vi "Plotting Main.vi"() -> ()   [LabVIEW 2016]
uses:
  Refrigeration/RTS/Type Definitions/RTS TDMS Filename Locations.ctl
panel:
  in  "TDMS Data Save":T1
  in  "Debug?":bool
  out "Debug array":string[](array[string])
  in  "Update Plot":bool
  out "Button":u16
  in  "OK":bool
  in  "Multicolumn Listbox":i32[](listbox)
  out "Mixed Signal Graph":T2(graph)
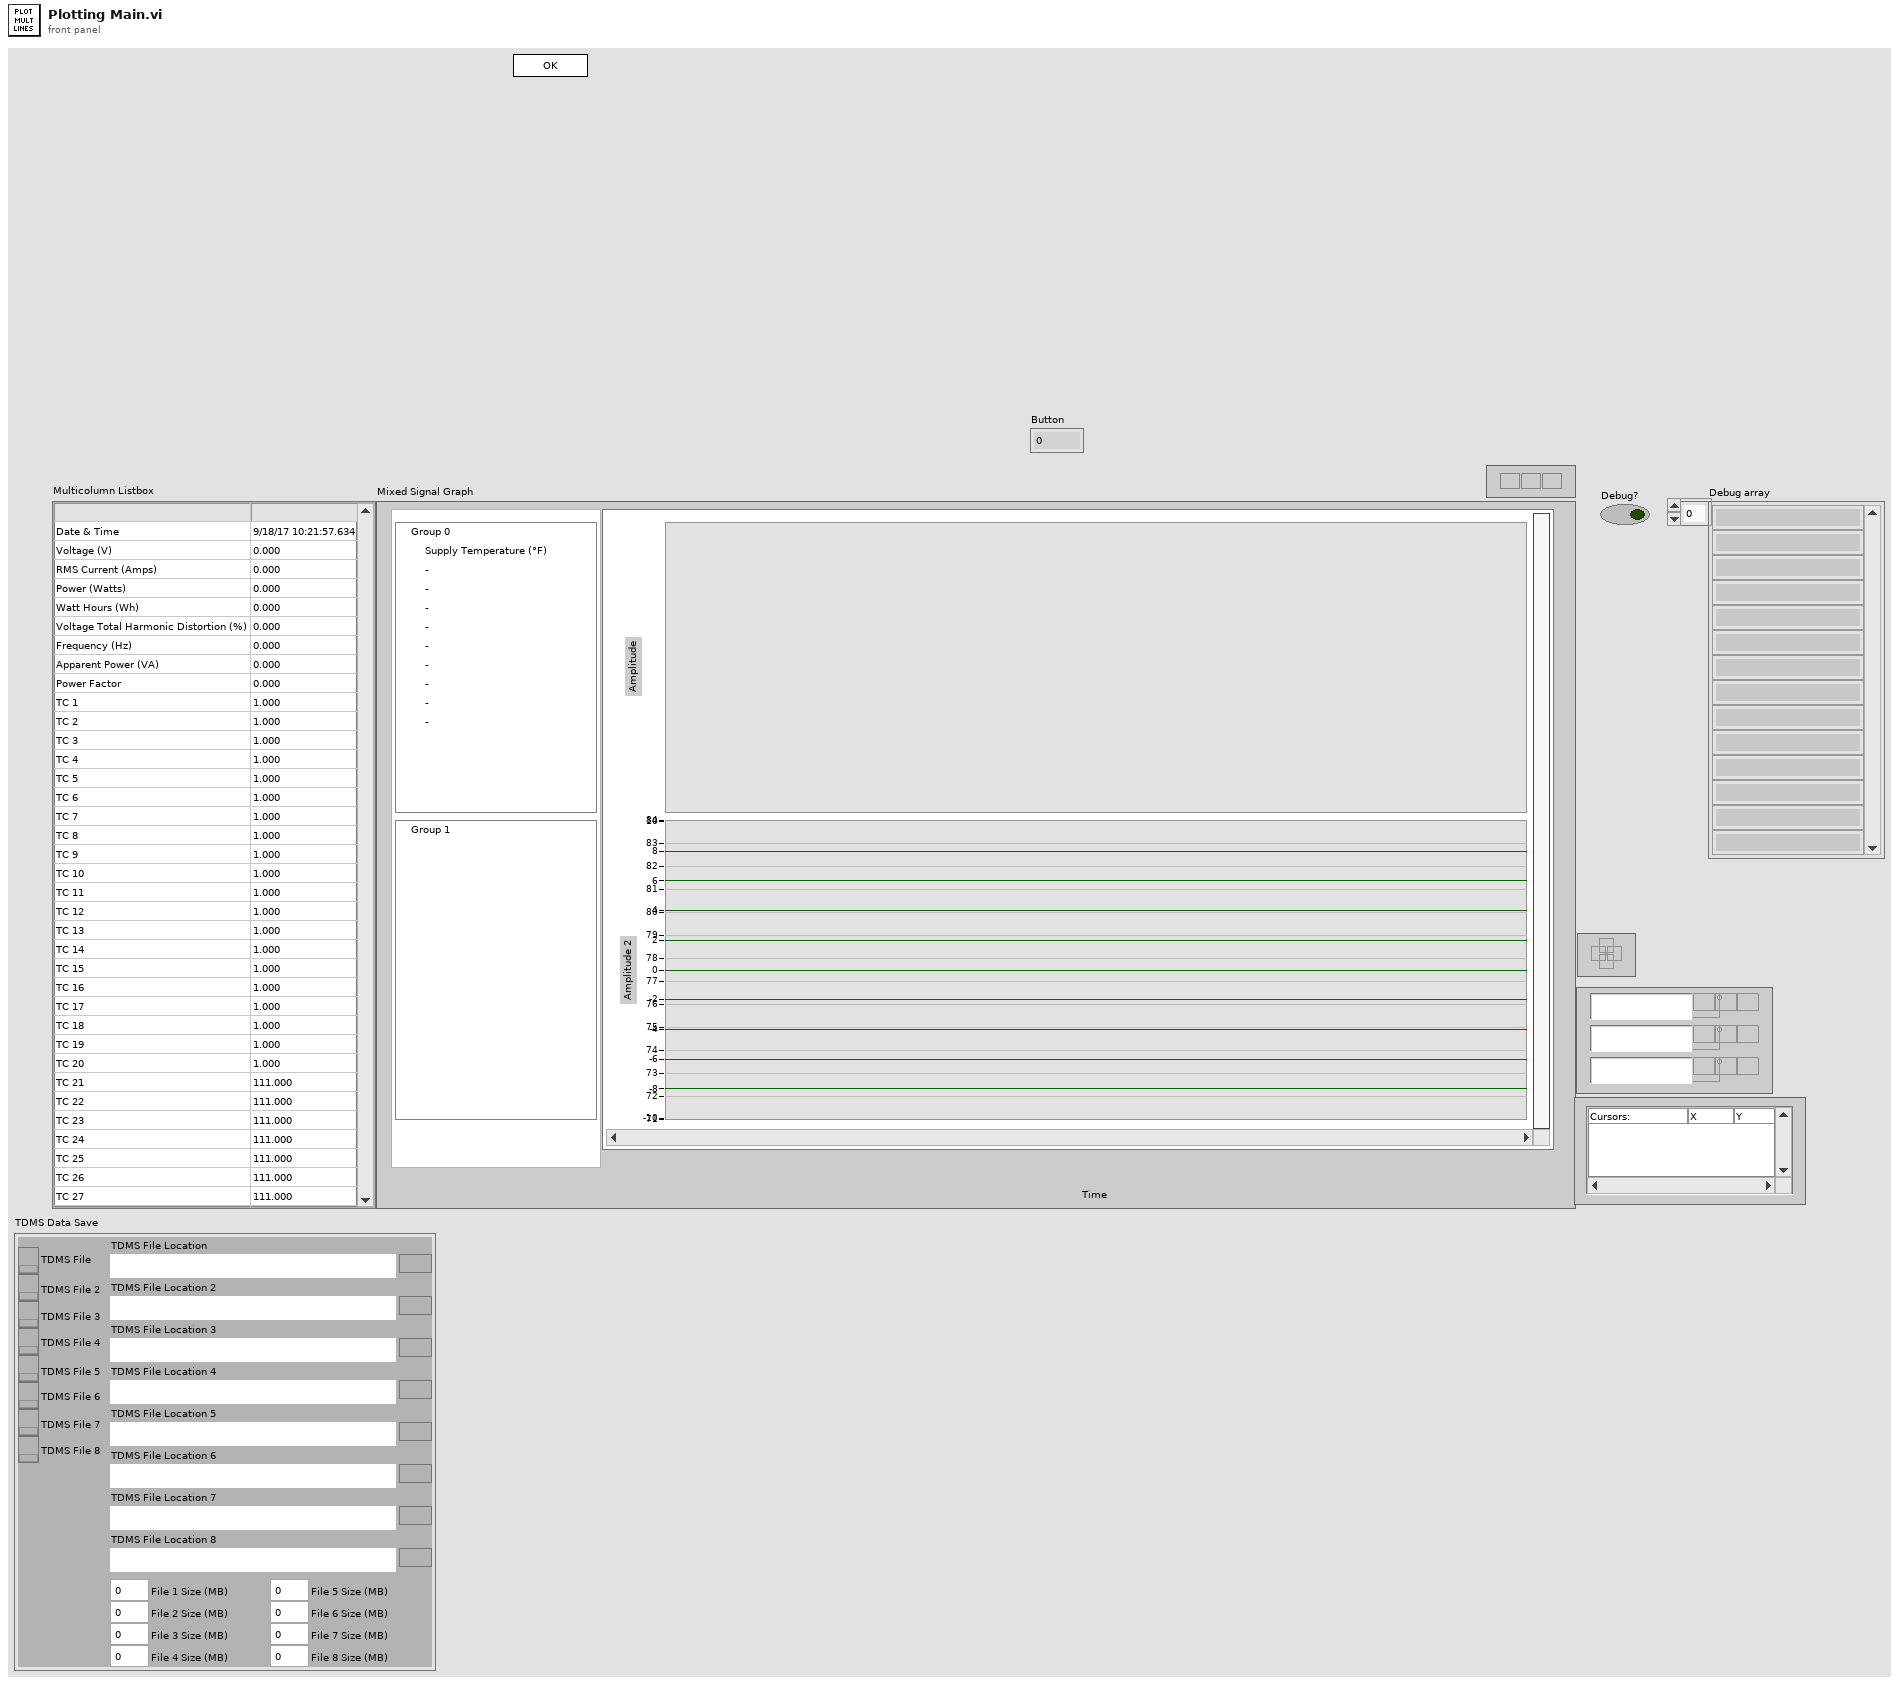
[diagram p1: front panel]
types:
  T1 = typedef "RTS TDMS Filename Locations.ctl" = cluster{"TDMS File":refnum<k34>, "TDMS File Location":path, "TDMS File Location 2":path, "TDMS File Location 3":path, "TDMS File Location 4":path, "TDMS File Location 5":path, "TDMS File Location 6":path, "TDMS File Location 7":path, "TDMS File Location 8":path, "TDMS File 2":refnum<k34>, "TDMS File 3":refnum<k34>, "TDMS File 4":refnum<k34>, "TDMS File 5":refnum<k34>, "TDMS File 6":refnum<k34>, "TDMS File 7":refnum<k34>, "TDMS File 8":refnum<k34>, "File 1 Size (MB)":dbl, "File 2 Size (MB)":dbl, "File 3 Size (MB)":dbl, "File 4 Size (MB)":dbl, "File 5 Size (MB)":dbl, "File 6 Size (MB)":dbl, "File 7 Size (MB)":dbl, "File 8 Size (MB)":dbl}
  T2 = cluster{"Waveform Graph":waveform(dbl), "Waveform Graph":waveform(dbl), "Waveform Graph":waveform(dbl), "Waveform Graph":waveform(dbl), "Waveform Graph":waveform(dbl), "Waveform Graph":waveform(dbl), "Waveform Graph":waveform(dbl), "Waveform Graph":waveform(dbl), "Waveform Graph":waveform(dbl), "Waveform Graph":waveform(dbl)}
  T3 = enum32{"invalid app kind", "Development System", "Run Time System", "Student Edition", "Embedded LabVIEW", "Evaluation", "Custom"}
  T4 = enum32{"Invalid", "Standard", "Closed", "Hidden", "Minimized", "Maximized"}
  T5 = cluster{"Core":cluster{"Current VI Reference":refnum<vi>, "Close Panel on Exit?":bool}, "ListBox Selection":i32[], "All Data":dbl[][], "Item Names":string[], "TDMS Data Save":T1}
  T6 = cluster{"Current VI Reference":refnum<vi>, "Close Panel on Exit?":bool}
  T7 = typedef "RTS TDMS Data.ctl" = cluster{"Station 1":dbl[][], "Station 2":dbl[][], "Station 3":dbl[][], "Station 4":dbl[][], "Station 5":dbl[][], "Station 6":dbl[][], "Station 7":dbl[][], "Station 8":dbl[][]}
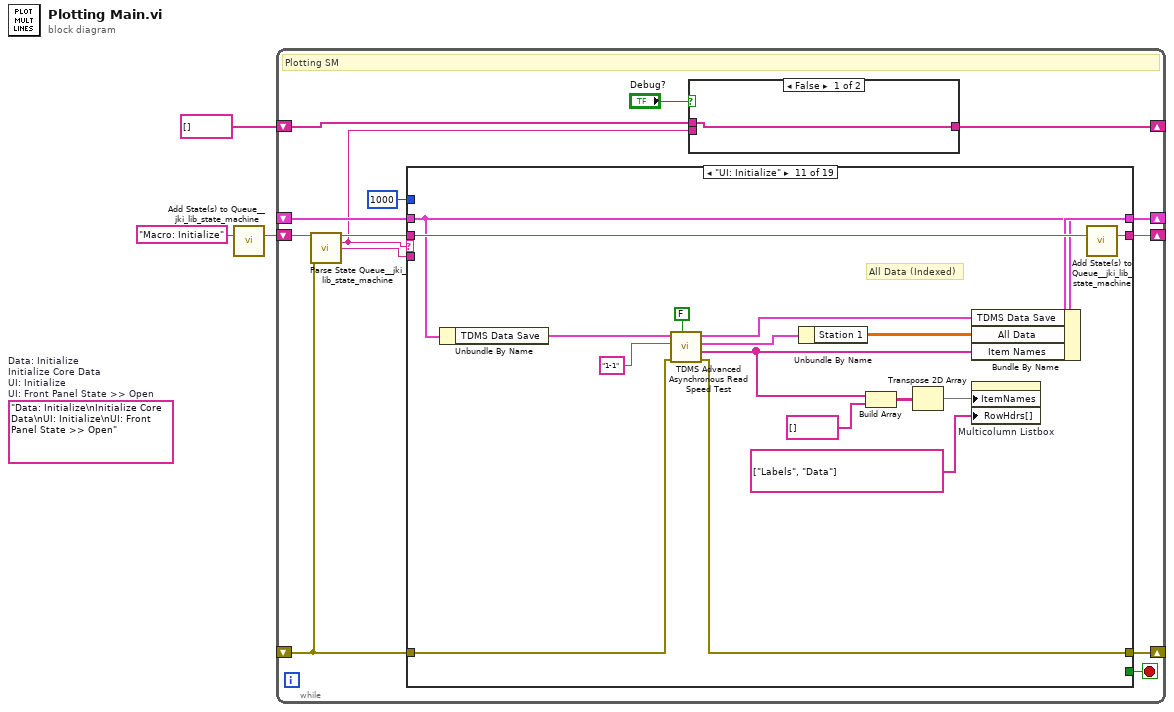
[diagram p0: block diagram]
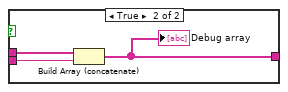
[diagram p2: hidden frame]
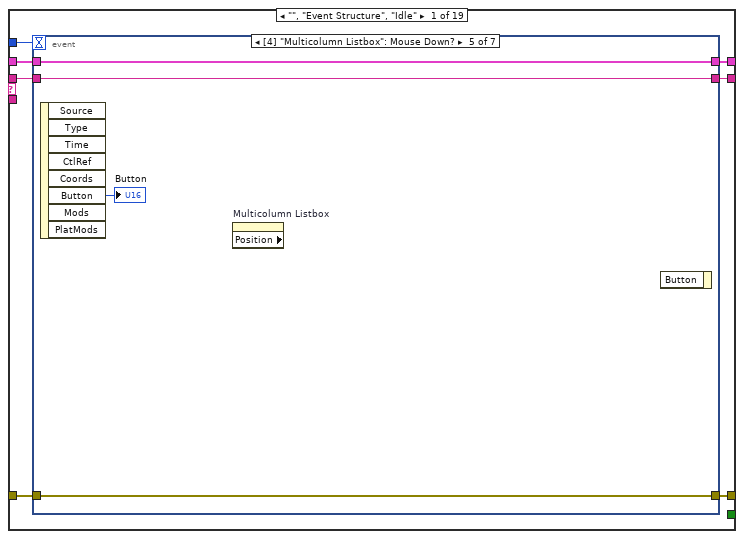
[diagram p3: hidden frame]
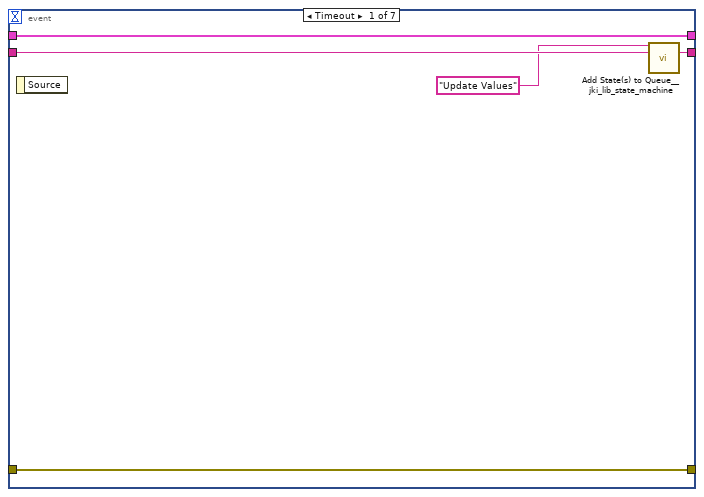
[diagram p4: hidden frame]
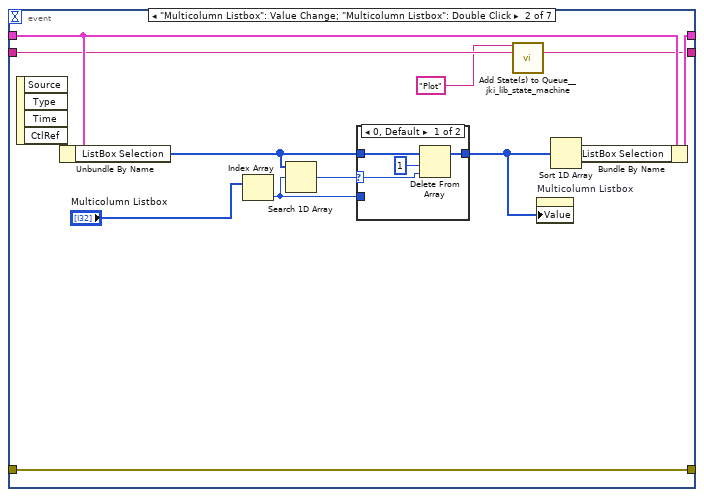
[diagram p5: hidden frame]
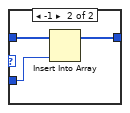
[diagram p6: hidden frame]
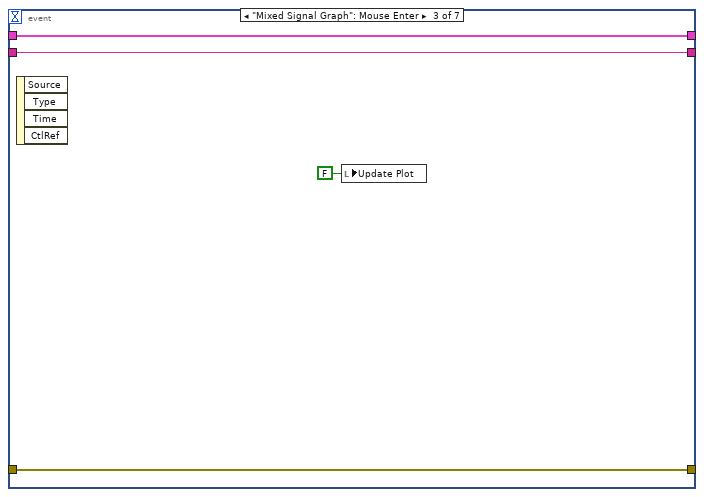
[diagram p7: hidden frame]
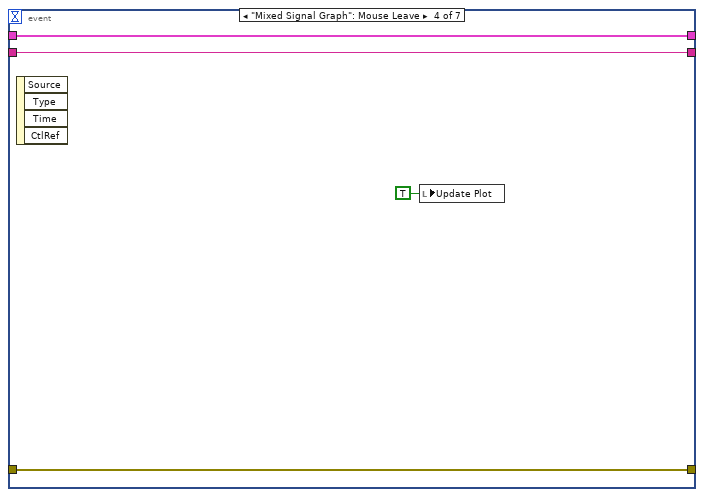
[diagram p8: hidden frame]
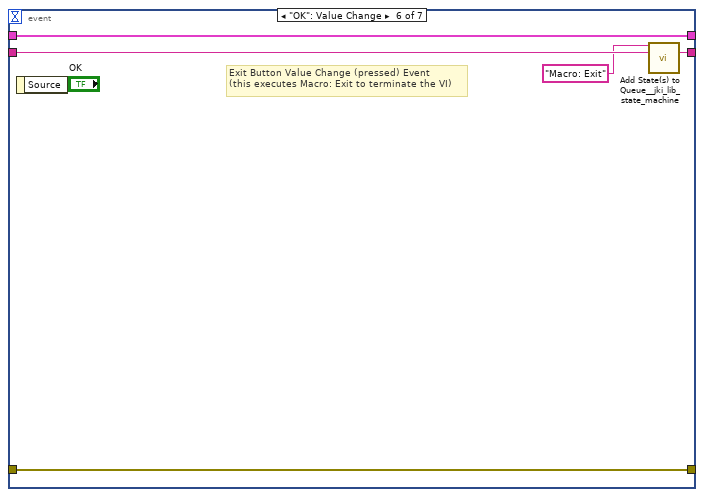
[diagram p9: hidden frame]
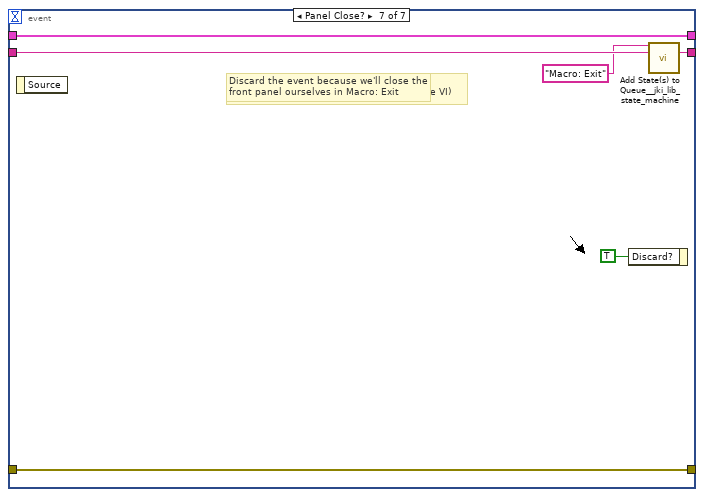
[diagram p10: hidden frame]
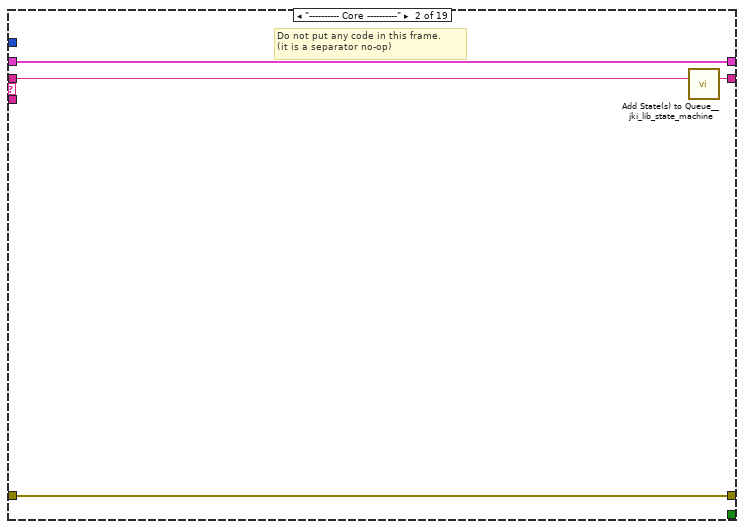
[diagram p11: hidden frame]
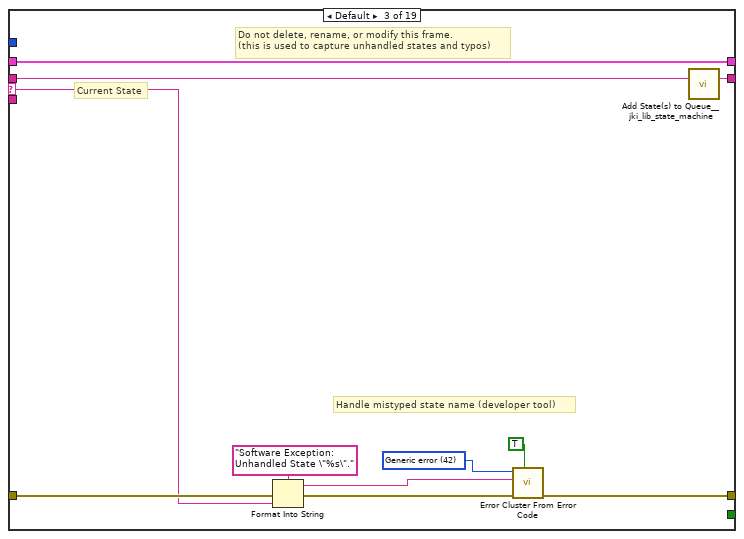
[diagram p12: hidden frame]
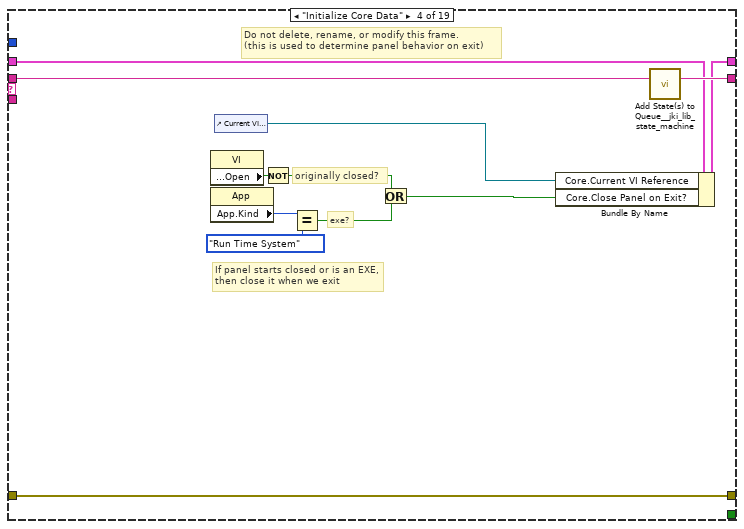
[diagram p13: hidden frame]
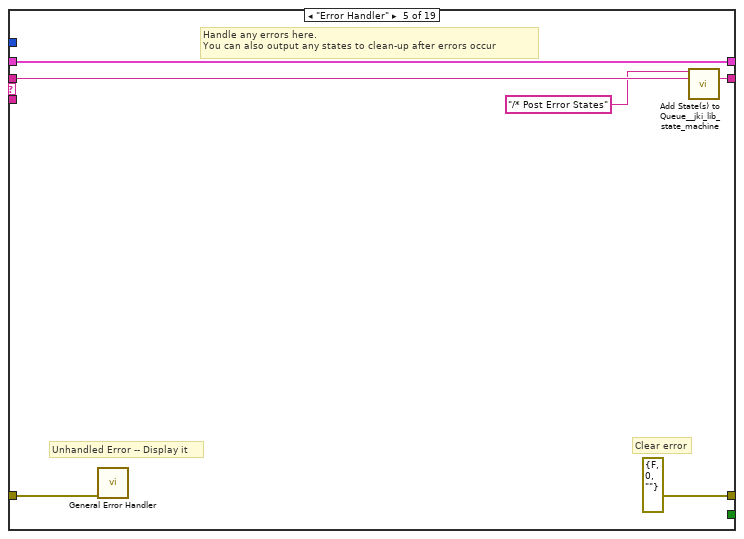
[diagram p14: hidden frame]
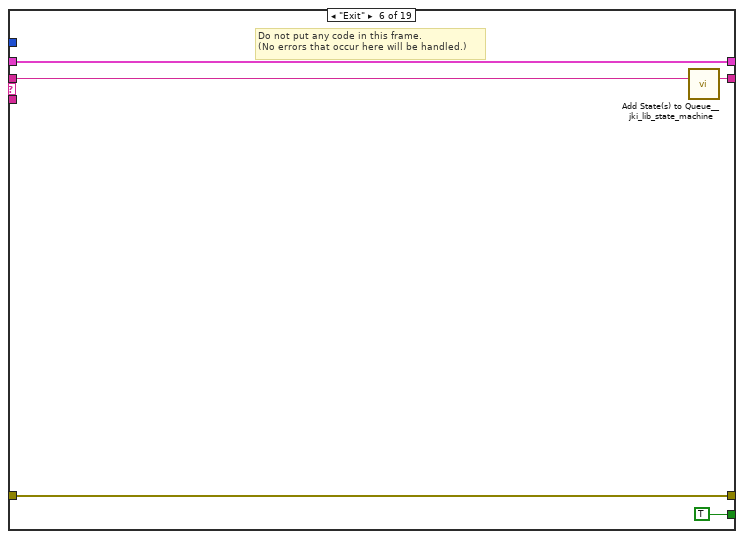
[diagram p15: hidden frame]
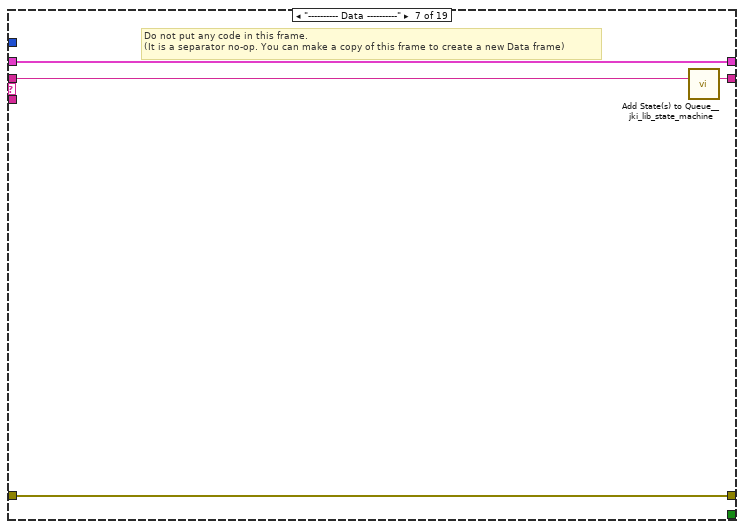
[diagram p16: hidden frame]
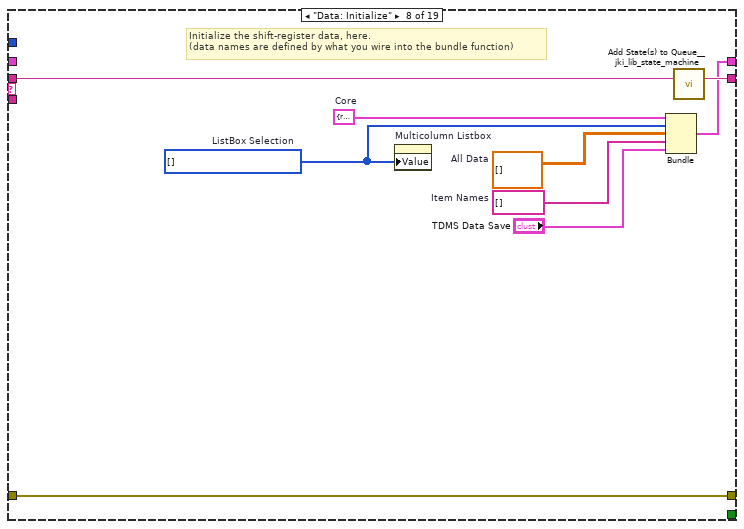
[diagram p17: hidden frame]
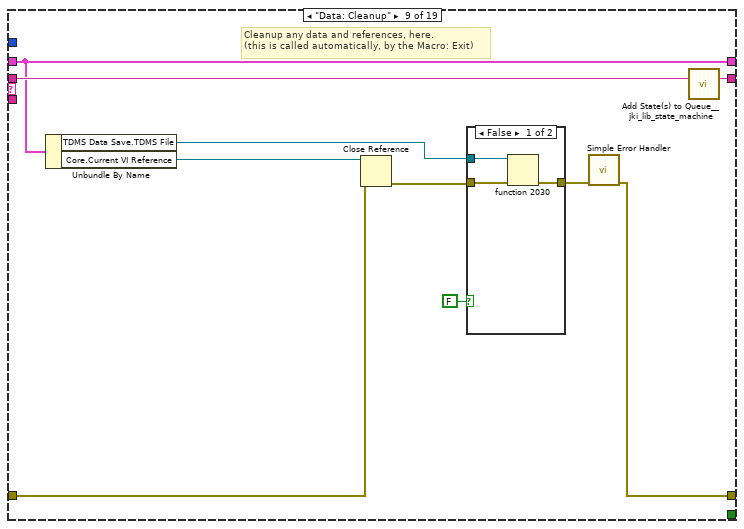
[diagram p18: hidden frame]
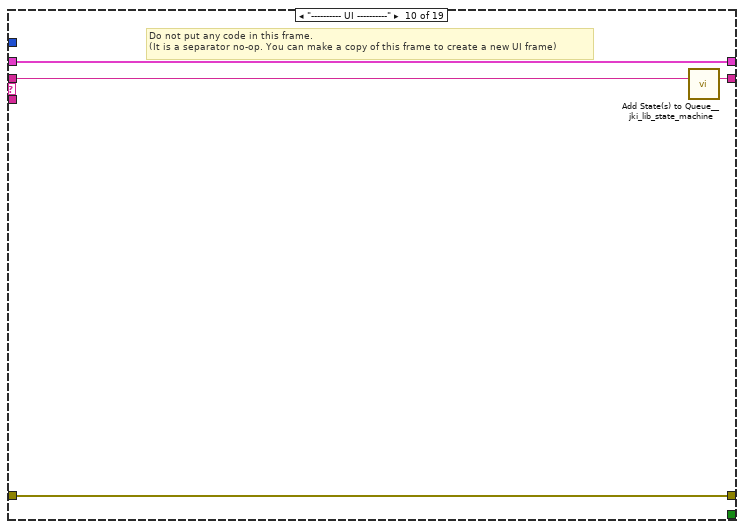
[diagram p20: hidden frame]
diagram:
  (unwired) "Data: Initialize\nInitialize Core Data\nUI: Initialize\nUI: Front Panel State >> Open"  # Data: Initialize Initialize Core Data UI: Initialize UI: Front Panel State >> Open
  n1 = call <vilib>:"Add State(s) to Queue__jki_lib_state_machine.vi"("State(s) in (\"\")"="Macro: Initialize") -> ("States Out"=w3:string)  [unwired: 14 in]
  n2 = while "Plotting SM" {
    shift-right: [w11] -> _
    shift-left: _ -> [w10]
    shift-right: [w14] -> _
    shift-left: _ -> [w8]
    shift-right: [w13] -> _
    shift-left: w3 -> [w15]
    shift-right: [w5] -> _
    shift-left: string[] [] -> [w7]
    stop <- w12 stop-if-true
    # "Plotting SM"
    n3 = call <vilib>:"Parse State Queue__jki_lib_state_machine.vi"("State Queue"=w15, "Error In (no error)"=w8) -> ("Remaining States"=w17:string, "Current State"=w6:string, "Arguments"=w16:string)  [unwired: 11 in]
    n4 = case shown="\"UI: Initialize\"" w6 {
      selector: w6 -> [_ _ w80 _ _ _ _ _ _ _ _ _ _ _ _ _ _ _ _]
      tunnel: w17 -> [w28 w79 w84 w102 w108 w113 w117 w126 w136 w144 w161 w167 w178 w204 w209 w219 w223 w231 w253]
      tunnel: w16 -> [_ _ _ _ _ _ _ _ _ _ _ w162 w172 _ _ _ _ _ _]
      tunnel: w10 -> [w26 w76 w82 w93 w105 w111 w114 _ w132 w141 w153 w165 w174 w201 w206 w216 w220 w228 w236]
      tunnel: [w25 w77 w86 w99 errorcluster {"status"=FALSE, "code"=0, "source"=""} ("error out") w110 w115 w123 w129 w142 w145 w163 w175 w202 w207 w217 w221 w229 w237] -> w14
      tunnel: w8 -> [w24 w77 w85 w99 w104 w110 w115 w123 w133 w142 w146 w164 w176 w202 w207 w217 w221 w229 w247]
      tunnel: [w27 w78 w83 w101 w107 w112 w116 w125 w135 w143 w160 w166 w177 w203 w208 w218 w222 w230 w252] -> w13
      tunnel: [_ _ _ _ _ TRUE _ _ _ _ _ _ _ _ _ _ _ _ _] -> w12
      tunnel: [w23 w76 w82 w100 w105 w111 w114 w124 w132 w141 w159 w165 w174 w201 w206 w216 w220 w228 w250] -> w11
      tunnel: 1000 ("Timeout") -> [w22 _ _ _ _ _ _ _ _ _ _ _ _ _ _ _ _ _ _]
      frame "", "Event Structure", "Idle" {
        n5 = event shown="[4] \"Multicolumn Listbox\": Mouse Down?" {
          selector: _ -> [_ _ _ _ _ _ _]
          dyn-events: _ -> [_ _ _ _ _ _ _]
          timeout: w22 -> [_ _ _ _ _ _ _]
          tunnel: w28 -> [w33 w38 w55 w59 w62 w69 w75]
          tunnel: [w32 w37 w55 w59 w62 w68 w74] -> w27
          tunnel: w26 -> [w30 w44 w56 w58 w63 w66 w72]
          tunnel: [w31 w45 w54 w60 w64 w67 w73] -> w25
          tunnel: w24 -> [w31 w45 w54 w60 w64 w67 w73]
          tunnel: [w30 w43 w56 w58 w63 w66 w72] -> w23
          event Timeout {
            n6 = event-data() -> ()  [unwired: 1 in, 1 out]
            n7 = call <vilib>:"Add State(s) to Queue__jki_lib_state_machine.vi"("State(s) in Front (\"\")"="Update Values" ("State(s) in Front (\"\")"), "State(s) in (\"\")"=w33) -> ("States Out"=w32:string)  [unwired: 13 in]
          }
          event "Multicolumn Listbox": Value Change; "Multicolumn Listbox": Double Click {
            n8 = event-data() -> ()  [unwired: 1 in, 4 out]
            n9 = Unbundle By Name(w44) -> ("ListBox Selection"=w39:i32[])
            n10 = Index Array(array="Multicolumn Listbox") -> (element=w41:i32)  [unwired: 1 in]
            n11 = Search 1D Array(1D array=w39, element=w41) -> (index of element=w40:i32)  [unwired: 1 in]
            n12 = case shown="0, Default" w40 {
              selector: w40 -> [w46 _]
              tunnel: w41 -> [_ w52]
              tunnel: w39 -> [w49 w51]
              tunnel: [w48 w50] -> w35
              frame 0, Default {
                n13 = Delete From Array(array=w49, length=1, index=w46) -> (array with subset deleted=w48:i32[])  [unwired: 1 out]
              }
              frame -1 {
                n14 = Insert Into Array(array=w51, new element=w52) -> (w50:i32[])  [unwired: 1 in]
              }
            }
            n15 = call <vilib>:"Add State(s) to Queue__jki_lib_state_machine.vi"("State(s) in Front (\"\")"="Plot" ("State(s) in Front (\"\")"), "State(s) in (\"\")"=w38) -> ("States Out"=w37:string)  [unwired: 13 in]
            n16 = property on="Multicolumn Listbox" class="MCListbox (strict)"("Value"=w35) -> ()  [unwired: 2 in, 2 out]
            n17 = Sort 1D Array(array=w35) -> (sorted array=w34:i32[])
            n18 = Bundle By Name(cluster=w44, "ListBox Selection"=w34) -> (w43:T5)
          }
          event "Mixed Signal Graph": Mouse Enter {
            n19 = event-data() -> ()  [unwired: 1 in, 4 out]
            n20 = local write "Update Plot"(FALSE ("Update Plot")) -> ()
          }
          event "Mixed Signal Graph": Mouse Leave {
            n21 = event-data() -> ()  [unwired: 1 in, 4 out]
            n22 = local write "Update Plot"(TRUE ("Update Plot")) -> ()
          }
          event "Multicolumn Listbox": Mouse Down? {
            n23 = event-data() -> ("Button"=→"Button":u16)  [unwired: 1 in, 7 out]
            n24 = property on="Multicolumn Listbox" class="MCListbox (strict)" props=["Position"]() -> ()  [unwired: 2 in, 3 out]
            n25 = event-data() -> ()  [unwired: 2 in, 1 out]
          }
          event "OK": Value Change {
            # "Exit Button Value Change (pressed) Event\n(this executes Macro: Exit to terminate the VI)"
            n26 = event-data() -> ()  [unwired: 1 in, 1 out]
            n27 = call <vilib>:"Add State(s) to Queue__jki_lib_state_machine.vi"("State(s) in Front (\"\")"="Macro: Exit", "State(s) in (\"\")"=w69) -> ("States Out"=w68:string)  [unwired: 13 in]
          }
          event Panel Close? {
            # "Discard the event because we'll close the front panel ourselves in Macro: Exit"
            # "Close Panel button (pressed) Event\n(this executes Macro: Exit to terminate the VI)"
            n28 = event-data() -> ()  [unwired: 1 in, 1 out]
            n29 = event-data("Discard?"=TRUE) -> ()  [unwired: 1 in, 1 out]
            n30 = call <vilib>:"Add State(s) to Queue__jki_lib_state_machine.vi"("State(s) in Front (\"\")"="Macro: Exit", "State(s) in (\"\")"=w75) -> ("States Out"=w74:string)  [unwired: 13 in]
          }
        }
      }
      frame "---------- Core ----------" {
        # "Do not put any code in this frame.\n(it is a separator no-op)"
        n31 = call <vilib>:"Add State(s) to Queue__jki_lib_state_machine.vi"("State(s) in (\"\")"=w79) -> ("States Out"=w78:string)  [unwired: 14 in]
      }
      frame Default {
        w89 = 42 items=["No error", "Argument error", "Memory is full", "Out of zone", "End of file", "File already open", "Generic file I/O error", "File not found", "File permission error", "Disk is full", "Duplicate path", "Too many files open", "System feature not enabled", "Resource file not found", "Cannot add resource", "Resource not found", "Image not found", "Image memory error", "Pen does not exist", "Config type invalid", "Config token not found", "Config parse error", "Config memory error", "Bad external code format", "Bad external code offset", "External code not present", "Null window", "Destroy window error", "Null menu", "Print aborted", "Bad print record", "Print driver error", "Windows error during printing", "Memory error during printing", "Print dialog error", "Generic print error", "Invalid device refnum", "Device not found", "Device parameter error", "Device unit error", "Cannot open device", "Device call aborted", "Generic error", "Cancelled by user", "Object ID too low", "Object ID too high", "Object not in heap", "Unknown heap", "Unknown object (invalid DefProc)", "Unknown object (DefProc not in table)", "Message out of range", "Invalid (null) method", "Unknown message", "Manager call not supported", "Bad address", "Network operation in progress", "Network operation timed out", "Connection is busy", "Network attribute not supported", "Network error", "Address in use", "System out of memory", "Connection aborted", "Connection refused", "Not connected", "Already connected", "Connection closed", "Initialization error (interapplication manager)", "Bad occurrence", "Wait on unbound occurrence handler", "Occurrence queue overflow", "Datalog type conflict", "Unused", "Unrecognized type (interapplication manager)", "Memory corrupt", "Failed to make temporary DLL", "Old CIN version", "Drag socket not found", "Failed to load drop-object", "Failed to register OLE object", "Failed to release OLE object", "Format specifier type mismatch", "Unknown format specifier", "Too few format specifiers", "Too many format specifiers", "Scan failed", "Newer CIN version", "Error converting to variant", "Runtime menu error", "Password tampered", "Variant attribute not found", "Incompatible variant data type", "Event data is not available", "Event Store is not present", "Occurrence is not found", "Event Queue is not created", "Event info is not available", "Refnum passed is NULL", "Error retrieving Class GUID", "Error retrieving CoClass GUID", "Error retrieving TypeLib GUID.", "Bad built application magic bytes.", "Specific driver is different from the specific driver associated with the Logical Name.", "There is no session opened to the class driver.", "Max Error", "MAX - Error with config objects", "MAX - Error loading configuration", "MAX - Group not supported"]
        # "Current State"
        # "Do not delete, rename, or modify this frame.\n(this is used to capture unhandled states and typos)"
        # "Handle mistyped state name (developer tool)"
        n32 = Format Into String(format string="Software Exception: Unhandled State \"%s\"." ("message"), error in=w85, w80) -> (resulting string=w88:string, error out=w87:errorcluster)  [unwired: 1 in]
        n33 = call <vilib>:"Error Cluster From Error Code.vi"("show call chain? (False)"=TRUE, "error in (no error)"=w87, "error message (\"\")"=w88, "error code (0)"=w89) -> ("error out"=w86:errorcluster)  [unwired: 5 in]
        n34 = call <vilib>:"Add State(s) to Queue__jki_lib_state_machine.vi"("State(s) in (\"\")"=w84) -> ("States Out"=w83:string)  [unwired: 14 in]
      }
      frame "Initialize Core Data" {
        # "Do not delete, rename, or modify this frame.\n(this is used to determine panel behavior on exit)"
        # "originally closed?"
        # "exe?"
        # "If panel starts closed or is an EXE, then close it when we exit"
        n35 = property class="VI"() -> ("Front Panel.Open"=w98:bool)  [unwired: 2 in, 2 out]
        n36 = property class="App"() -> ("App.Kind"=w97:T3)  [unwired: 2 in, 2 out]
        n37 = control-ref of="Current VI Reference"() -> (w91:refnum<vi>)
        n38 = Not(x=w98) -> (.not. x?=w95:bool)
        n39 = Equal?(x=w97, y=T3."Run Time System" ("Application:Kind")) -> (x = y?=w94:bool)
        n40 = Or(x=w95, y=w94) -> (x .or. y?=w92:bool)
        n41 = Bundle By Name(cluster=w93, "Core.Current VI Reference"=w91, "Core.Close Panel on Exit?"=w92) -> (w100:T5)
        n42 = call <vilib>:"Add State(s) to Queue__jki_lib_state_machine.vi"("State(s) in (\"\")"=w102) -> ("States Out"=w101:string)  [unwired: 14 in]
      }
      frame "Error Handler" {
        # "Unhandled Error -- Display it"
        # "Handle any errors here.\nYou can also output any states to clean-up after errors occur"
        # "Clear error"
        n43 = call <vilib>:"General Error Handler.vi"("error in (no error)"=w104) -> ()  [unwired: 10 in, 5 out]
        n44 = call <vilib>:"Add State(s) to Queue__jki_lib_state_machine.vi"("State(s) in Front (\"\")"="/* Post Error States", "State(s) in (\"\")"=w108) -> ("States Out"=w107:string)  [unwired: 13 in]
      }
      frame "Exit" {
        # "Do not put any code in this frame.\n(No errors that occur here will be handled.)"
        n45 = call <vilib>:"Add State(s) to Queue__jki_lib_state_machine.vi"("State(s) in (\"\")"=w113) -> ("States Out"=w112:string)  [unwired: 14 in]
      }
      frame "---------- Data ----------" {
        # "Do not put any code in this frame.\n(It is a separator no-op. You can make a copy of this frame to create a new Data frame)"
        n46 = call <vilib>:"Add State(s) to Queue__jki_lib_state_machine.vi"("State(s) in (\"\")"=w117) -> ("States Out"=w116:string)  [unwired: 14 in]
      }
      frame "Data: Initialize" {
        w119 = string[] []  # Item Names
        w120 = dbl[][] []  # All Data
        w121 = i32[] []  # ListBox Selection
        w122 = T6 {"Current VI Reference"=refnum, "Close Panel on Exit?"=FALSE}  # Core
        # "Initialize the shift-register data, here.\n(data names are defined by what you wire into the bundle function)"
        n47 = property on="Multicolumn Listbox" class="MCListbox (strict)"("Value"=w121) -> ()  [unwired: 2 in, 2 out]
        n48 = Bundle("Core"=w122, "ListBox Selection"=w121, "All Data"=w120, "Item Names"=w119, "TDMS Data Save"="TDMS Data Save") -> (w124:T5)  [unwired: 1 in]
        n49 = call <vilib>:"Add State(s) to Queue__jki_lib_state_machine.vi"("State(s) in (\"\")"=w126) -> ("States Out"=w125:string)  [unwired: 14 in]
      }
      frame "Data: Cleanup" {
        # "Cleanup any data and references, here.\n(this is called automatically, by the Macro: Exit)"
        n50 = Unbundle By Name(w132) -> ("TDMS Data Save.TDMS File"=w127:refnum<k34>, "Core.Current VI Reference"=w134:refnum<vi>)
        n51 = Close Reference(reference=w134, error in (no error)=w133) -> (error out=w130:errorcluster)
        n52 = case shown="False" FALSE {
          tunnel: [w139 w140] -> w131
          tunnel: w127 -> [w138 _]
          tunnel: w130 -> [w137 w140]
          frame False {
            n53 = fn#2030(8:w137, 11:w138) -> (0:w139:errorcluster)  [unwired: 1 out]
          }
          frame True {
          }
        }
        n54 = call <vilib>:"Simple Error Handler.vi"("error in (no error)"=w131) -> ("error out"=w129:errorcluster)  [unwired: 1 in, 7 out]
        n55 = call <vilib>:"Add State(s) to Queue__jki_lib_state_machine.vi"("State(s) in (\"\")"=w136) -> ("States Out"=w135:string)  [unwired: 14 in]
      }
      frame "---------- UI ----------" {
        # "Do not put any code in this frame.\n(It is a separator no-op. You can make a copy of this frame to create a new UI frame)"
        n56 = call <vilib>:"Add State(s) to Queue__jki_lib_state_machine.vi"("State(s) in (\"\")"=w144) -> ("States Out"=w143:string)  [unwired: 14 in]
      }
      frame "UI: Initialize" {
        # "All Data (Indexed)"
        n57 = Unbundle By Name(w153) -> ("TDMS Data Save"=w147:T1)
        n58 = call "TDMS Advanced Asynchronous Read Speed Test.vi"("Debug"=FALSE, "Error In"=w146, "Tree Selection"="1-1" ("Station ID"), "TDMS Data Save"=w147) -> ("Error Out"=w145:errorcluster, "channel name(s) out"=w151:string[], "TDMS Data"=w150:T7, "TDMS Data Save Output"=w149:T1)  [unwired: 4 in]
        n59 = Unbundle By Name(w150) -> ("Station 1"=w154:dbl[][])
        n60 = Build Array(w151, string[] [] ("element")) -> (w157:string[][])
        n61 = Transpose 2D Array(2D array=w157) -> (transposed array=w156:string[][])
        n62 = Bundle By Name(cluster=w153, "TDMS Data Save"=w149, "All Data"=w154, "Item Names"=w151) -> (w159:T5)
        n63 = property on="Multicolumn Listbox" class="MCListbox (strict)"("ItemNames"=w156, "RowHdrs[]"=string[] ["Labels", "Data"] ("Row Header Strings[]")) -> ()  [unwired: 2 in, 2 out]
        n64 = call <vilib>:"Add State(s) to Queue__jki_lib_state_machine.vi"("State(s) in (\"\")"=w161) -> ("States Out"=w160:string)  [unwired: 14 in]
      }
      frame "UI: Cursor Set" {
        # "Argument"
        # "Set and Unset Cursor Busy.\n(Usage: \"UI: Cursor Set >> Busy|Idle\")"
        n65 = case shown="\"Idle\", Default" w162 {
          tunnel: w164 -> [w169 w171]
          tunnel: [w168 w170] -> w163
          frame "Idle", Default {
            n66 = call <vilib>:"Unset Busy.vi"("error in (no error)"=w169) -> ("error out"=w168:errorcluster)  [unwired: 10 in]
          }
          frame "Busy" {
            n67 = call <vilib>:"Set Busy.vi"("error in (no error)"=w171) -> ("error out"=w170:errorcluster)  [unwired: 9 in, 1 out]
          }
        }
        n68 = call <vilib>:"Add State(s) to Queue__jki_lib_state_machine.vi"("State(s) in (\"\")"=w167) -> ("States Out"=w166:string)  [unwired: 14 in]
      }
      frame "UI: Front Panel State" {
        # "Argument"
        # "Set Front Panel Open or Closed\n(Usage: \"UI: Front Panel State >> Open|Close\")"
        n69 = Unbundle By Name(w174) -> ("Core.Current VI Reference"=w173:refnum<vi>)
        n70 = case shown="\"Open\", Default" w172 {
          tunnel: w176 -> [w182 w195]
          tunnel: [w184 w196] -> w175
          tunnel: w173 -> [w183 w193]
          frame "Open", Default {
            n71 = property class="VI"(reference=w183, error in=w182) -> (reference out=w180:refnum<vi>, error out=w181:errorcluster, "Front Panel.Open"=w179:bool)
            n72 = case shown="True" w179 {
              tunnel: [w187 w190] -> w184
              tunnel: w181 -> [w186 w190]
              tunnel: w180 -> [w185 _]
              frame False {
                n73 = invoke class="VI" method="FP.Open"(reference=w185, error in=w186, "Activate"=TRUE, "State"=T4."Standard") -> (error out=w187:errorcluster)  [unwired: 1 in, 4 out]
              }
              frame True {
              }
            }
          }
          frame "Close" {
            n74 = property class="VI"(reference=w193, error in=w195) -> (reference out=w192:refnum<vi>, error out=w194:errorcluster, "Front Panel.Open"=w191:bool)
            n75 = case shown="True" w191 {
              tunnel: [w197 w200] -> w196
              tunnel: w194 -> [w197 w199]
              tunnel: w192 -> [_ w198]
              frame False {
              }
              frame True {
                n76 = invoke class="VI" method="FP.Close"(reference=w198, error in=w199) -> (error out=w200:errorcluster)  [unwired: 1 in, 2 out]
              }
            }
          }
        }
        n77 = call <vilib>:"Add State(s) to Queue__jki_lib_state_machine.vi"("State(s) in (\"\")"=w178) -> ("States Out"=w177:string)  [unwired: 14 in]
      }
      frame "---------- Macro ----------" {
        # "Do not put any code in this frame.\n(It is a separator no-op. You can make a copy of this frame to create a new Macro frame)"
        n78 = call <vilib>:"Add State(s) to Queue__jki_lib_state_machine.vi"("State(s) in (\"\")"=w204) -> ("States Out"=w203:string)  [unwired: 14 in]
      }
      frame "Macro: Initialize" {
        w205 = "Data: Initialize\nInitialize Core Data\nUI: Initialize\nUI: Front Panel State >> Open"  # Data: Initialize Initialize Core Data UI: Initialize UI: Front Panel State >> Open
        # "Initialization Macro\n(This is called once, when the VI starts)"
        n79 = call <vilib>:"Add State(s) to Queue__jki_lib_state_machine.vi"("State(s) in Front (\"\")"=w205, "State(s) in (\"\")"=w209) -> ("States Out"=w208:string)  [unwired: 13 in]
      }
      frame "Macro: Exit" {
        # "Exit Macro\n(This is called once, when the VI exits)"
        n80 = Unbundle By Name(w216) -> ("Core.Close Panel on Exit?"=w215:bool)
        n81 = Select(t="UI: Front Panel State >> Close", s=w215, f="") -> (s? t:f=w212:string)
        n82 = call <vilib>:"Add State(s) to Queue__jki_lib_state_machine.vi"("State(s) in (\"\")"=w212, "State(s) at Back (\"\")"="Data: Cleanup\nExit") -> ("States Out"=w210:string)  [unwired: 13 in]
        n83 = call <vilib>:"Add State(s) to Queue__jki_lib_state_machine.vi"("State(s) in Front (\"\")"=w210, "State(s) in (\"\")"=w219) -> ("States Out"=w218:string)  [unwired: 13 in]
      }
      frame "---------- New Category ----------" {
        # "Template Separator\n(You can make a copy of, or modify, this frame)"
        n84 = call <vilib>:"Add State(s) to Queue__jki_lib_state_machine.vi"("State(s) in (\"\")"=w223) -> ("States Out"=w222:string)  [unwired: 14 in]
      }
      frame "Plot" {
        n85 = Unbundle By Name(w228) -> ("All Data"=w224:dbl[][], "ListBox Selection"=w227:i32[], "Item Names"=w225:string[])
        n86 = call "Plotting Assemble.vi"("Item Names"=w225, "OldVal"=w227, "All Data"=w224) -> ("Mixed Signal Graph"=→"Mixed Signal Graph":T2)  [unwired: 8 in]
        n87 = call <vilib>:"Add State(s) to Queue__jki_lib_state_machine.vi"("State(s) in (\"\")"=w231) -> ("States Out"=w230:string)  [unwired: 14 in]
      }
      frame "Update Values" {
        n88 = Unbundle By Name(w236) -> ("All Data"=w235:dbl[][], "Item Names"=w234:string[], "TDMS Data Save"=w232:T1)
        n89 = call "RTS Get TDMS Data.vi"("Read All?"=FALSE, "Tree Selection"="1-1" ("Station ID"), "Debug"=FALSE, "error in (no error)"=w247, "TDMS Data Save"=w232) -> ("error out"=w238:errorcluster, "TDMS Data Output"=w246:T7, "TDMS Data Save Output"=w233:T1)  [unwired: 3 in, 1 out]
        n90 = Unbundle By Name(w246) -> ("Station 1"=w241:dbl[][])
        n91 = Index Array(array=w241, index (row)=0) -> (element=w239:dbl[])  [unwired: 1 in]
        n92 = case shown="True" "Update Plot" {
          tunnel: ["" ("State(s) in Front (\"\")") "Plot" ("State(s) in Front (\"\")")] -> w249
          frame False {
          }
          frame True {
          }
        }
        n93 = call "Plotting List Box Names.vi"("Error In"=w238, "Item Names"=w234, "Station 1"=w241) -> ("Error Out"=w237:errorcluster, "Listbox names"=w251:string[][])  [unwired: 6 in, 1 out]
        n94 = Build Array (concatenate)(w235, w239) -> (w242:dbl[][])
        n95 = property on="Multicolumn Listbox" class="MCListbox (strict)"("ItemNames"=w251) -> ()  [unwired: 2 in, 2 out]
        n96 = Bundle By Name(cluster=w236, "All Data"=w242, "TDMS Data Save"=w233) -> (w250:T5)
        n97 = call <vilib>:"Add State(s) to Queue__jki_lib_state_machine.vi"("State(s) in Front (\"\")"=w249, "State(s) in (\"\")"=w253) -> ("States Out"=w252:string)  [unwired: 13 in]
      }
    }
    n98 = case shown="False" "Debug?" {
      tunnel: w7 -> [w18 w21]
      tunnel: w6 -> [_ w20]
      tunnel: [w18 w19] -> w5
      frame False {
      }
      frame True {
        n99 = Build Array (concatenate)(w21, w20) -> (w19:string[])
        "Debug array" <- w19
      }
    }
  }
